vi "file_interative_manager.vi"() -> ()   [LabVIEW 2014]
uses:
  machine_ops/machine.lvclass
panel:
  in  "input_machine_reference.lvclass":refnum<class "machine.lvclass">
  in  "save_file_type":T1(ring)
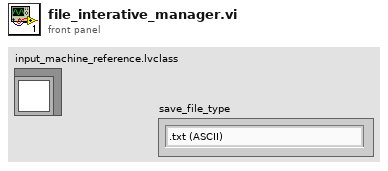
[diagram p1: front panel]
types:
  T1 = enum16{".txt (ASCII)", ".csv (ASCII)", ".xls (ASCII)"}
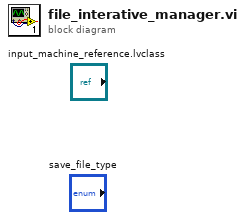
[diagram p0: block diagram]
diagram:
